vi "JoystickInput.vi"(11 "JoystickDevRef":T2) -> (1 "Buttons":bool[](array[boolean]), 2 "Axes":dbl[](array[numeric]), 3 "output cluster":T1, 4 "POVs":i16[](array[numeric]))   [LabVIEW 2017]
uses:
  <vilib>/Rock Robotics/WPI/Joystick/WPI_JoystickDevRef.ctl
  <vilib>/Rock Robotics/WPI/Joystick/WPI_JoystickDeviceEnum.ctl
panel:
  out "Generic_Buttons":bool[](array[boolean])
  out "Generic_Axes":dbl[](array[numeric])
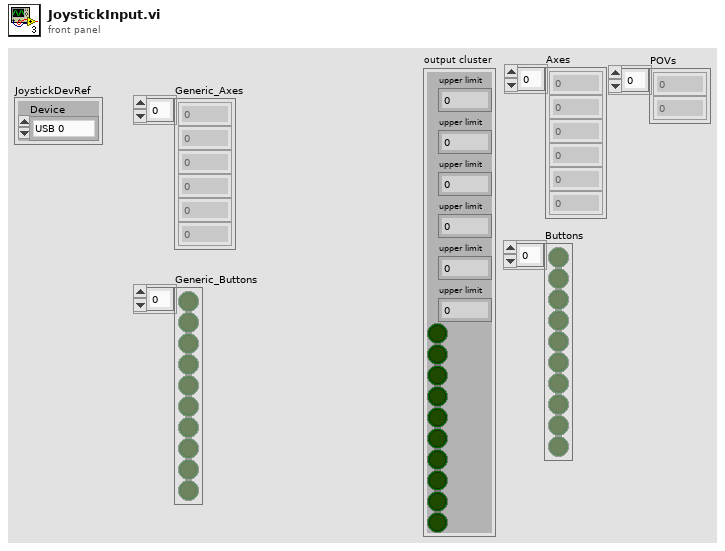
[diagram p1: front panel]
types:
  T1 = cluster{"upper limit":dbl, "upper limit":dbl, "upper limit":dbl, "upper limit":dbl, "upper limit":dbl, "upper limit":dbl, bool, bool, bool, bool, bool, bool, bool, bool, bool, bool}
  T2 = typedef "WPI_JoystickDevRef.ctl" = cluster{"Device":T3}
  T3 = typedef "WPI_JoystickDeviceEnum.ctl" = enum16{"USB 0", "USB 1", "USB 2", "USB 3", "USB 4", "USB 5"}
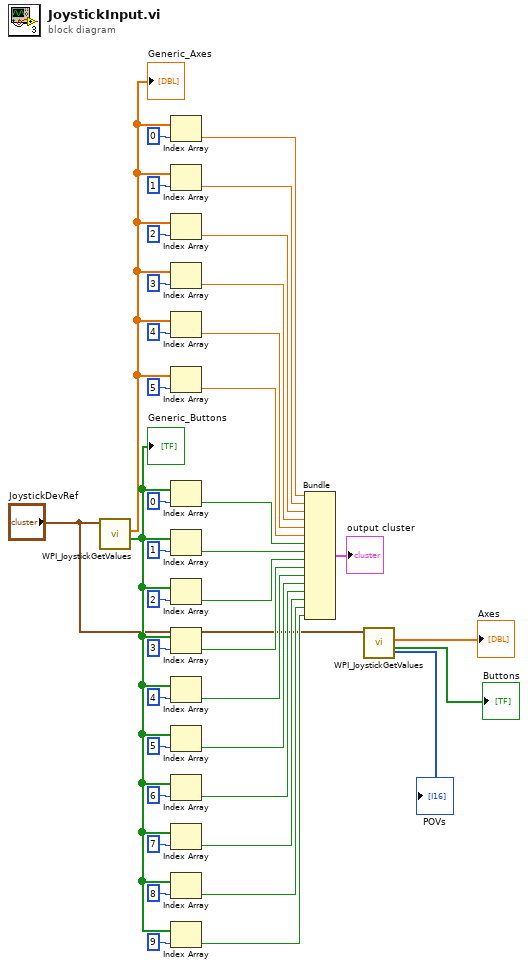
[diagram p0: block diagram]
diagram:
  n1 = call <vilib>:"WPI_JoystickGetValues.vi"("JoystickDevRef"="JoystickDevRef") -> ("Buttons"=w29:bool[], "Axes"=w22:dbl[])  [unwired: 6 in, 3 out]
  "Generic_Axes" <- w22
  "Generic_Buttons" <- w29
  n2 = Index Array(array=w22, index=0) -> (element=w21:dbl)
  n3 = Index Array(array=w22, index=1) -> (element=w20:dbl)
  n4 = Index Array(array=w22, index=2) -> (element=w19:dbl)
  n5 = Index Array(array=w22, index=3) -> (element=w18:dbl)
  n6 = Index Array(array=w22, index=4) -> (element=w17:dbl)
  n7 = Index Array(array=w22, index=5) -> (element=w16:dbl)
  n8 = Index Array(array=w29, index=0) -> (element=w15:bool)
  n9 = Index Array(array=w29, index=1) -> (element=w14:bool)
  n10 = Index Array(array=w29, index=2) -> (element=w13:bool)
  n11 = Index Array(array=w29, index=3) -> (element=w12:bool)
  n12 = Index Array(array=w29, index=4) -> (element=w11:bool)
  n13 = Index Array(array=w29, index=5) -> (element=w10:bool)
  n14 = Index Array(array=w29, index=6) -> (element=w9:bool)
  n15 = Index Array(array=w29, index=7) -> (element=w8:bool)
  n16 = Index Array(array=w29, index=8) -> (element=w7:bool)
  n17 = Index Array(array=w29, index=9) -> (element=w6:bool)
  n18 = Bundle("upper limit"=w21, "upper limit"=w20, "upper limit"=w19, "upper limit"=w18, "upper limit"=w17, "upper limit"=w16, w15, w14, w13, w12, w11, w10, w9, w8, w7, w6) -> (→"output cluster":T1)  [unwired: 1 in]
  n19 = call <vilib>:"WPI_JoystickGetValues.vi"("JoystickDevRef"="JoystickDevRef") -> ("Buttons"=→"Buttons":bool[], "Axes"=→"Axes":dbl[], "POVs"=→"POVs":i16[])  [unwired: 6 in, 2 out]
